vi "template.vi"(8 "error in":errorcluster, 11 "object_in":cluster{"handle":i32}) -> (0 "error out":errorcluster, 3 "object_out":dbl)   [LabVIEW 2020]
uses:
  <vilib>/Utility/file.llb/Write Delimited Spreadsheet (DBL).vi
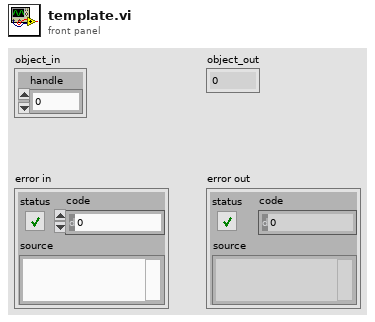
[diagram p1: front panel]
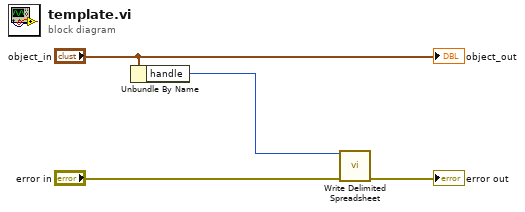
[diagram p0: block diagram]
diagram:
  n1 = Unbundle By Name("object_in") -> ("handle"=w2:i32)
  n2 = call-poly <vilib>:"Write Delimited Spreadsheet.vi"("file path (dialog if empty)"=w2, "error in (no error)"="error in") -> ("error out"=→"error out":errorcluster)  [unwired: 12 in, 1 out]
  "object_out" <- "object_in"
